vi "setClusterElement.vi"(8 "error in (no error)":errorcluster, 9 "Value":variant, 10 "Label.Text":string, 11 "reference":refnum<vi>) -> (0 "error out":errorcluster, 3 "reference 2":refnum<vi>)   [LabVIEW 2014]
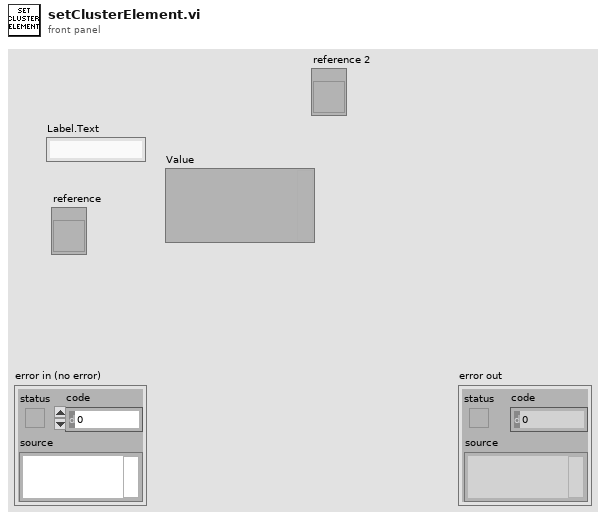
[diagram p1: front panel]
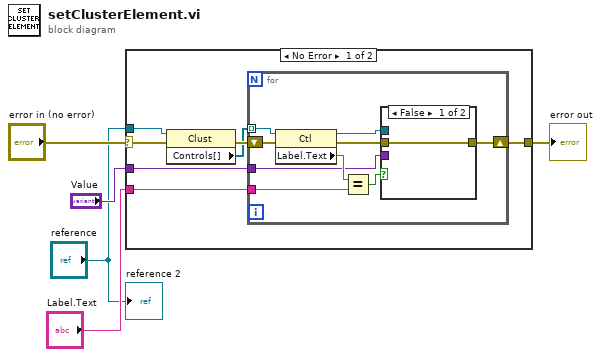
[diagram p0: block diagram]
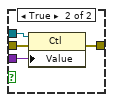
[diagram p2: hidden frame]
diagram:
  n1 = case shown="No Error" "error in (no error)" {
    selector: "error in (no error)" -> [w10 w27]
    tunnel: [w9 w27] -> w4
    tunnel: "reference" -> [w8 _]
    tunnel: "Label.Text" -> [w7 _]
    tunnel: "Value" -> [w6 _]
    frame No Error {
      n2 = property class="Clust"(reference=w8, error in=w10) -> (error out=w12:errorcluster, "Controls[]"=w11:refnum<vi>[])  [unwired: 1 out]
      n3 = for {
        shift-right: [w13] -> w9
        shift-left: w12 -> [w21]
        tunnel: w11 -> [w20] mode=indexing
        tunnel: w7 -> [w17]
        tunnel: w6 -> [w14]
        n4 = property class="Ctl"(reference=w20, error in=w21) -> (reference out=w15:refnum<vi>, error out=w19:errorcluster, "Label.Text"=w18:string)
        n5 = Equal?(x=w18, y=w17) -> (x = y?=w16:bool)
        n6 = case shown="False" w16 {
          tunnel: w19 -> [w22 w24]
          tunnel: w15 -> [_ w26]
          tunnel: w14 -> [_ w25]
          tunnel: [w22 w23] -> w13
          frame False {
          }
          frame True {
            n7 = property class="Ctl"(reference=w26, error in=w24, "Value"=w25) -> (error out=w23:errorcluster)  [unwired: 1 out]
          }
        }
      }
    }
    frame Error {
    }
  }
  "error out" <- w4
  "reference 2" <- "reference"
